vi "Init.vi"(8 "error in (no error)":errorcluster, 10 "Address":string, 11 "BPC30x in":refnum<class "BPC30x.lvclass">) -> (0 "error out":errorcluster, 3 "BPC30x out":refnum<class "BPC30x.lvclass">)   [LabVIEW 2023, in "BPC30x.lvlib" / "BPC30x.lvclass"]
uses:
  BPC30x.lvclass
  C:/Users/quantum/Documents/LVDAQ/UIs/TranslationStage_UI/Thorlabs.MotionControl.Controls.dll
  UIs/TranslationStage_UI/Thorlabs.MotionControl.Controls.dll
  typedefs/instrumentType.ctl
  typedefs/typedefs.lvlib
  <vilib>/ActorFramework/Actor/Actor.lvclass
  Interfaces/InitDeinitInterface/InitDeinitComm Messages/InitDone Msg/InitDone Msg.lvclass
  C:/Program Files/National Instruments/LabVIEW 2023/vi.lib/ActorFramework/Actor/Actor.lvclass
  C:/Users/quantum/Documents/LVDAQ/ConcreteClasses/ConcreteInstrumentClasses/BPC301/BPC30x/BPC30x.lvclass
  C:/Users/quantum/Documents/LVDAQ/Interfaces/InitDeinitInterface/InitDeinit/InitDeinit.lvclass
  C:/Users/quantum/Documents/LVDAQ/Interfaces/AbstractInstrumentClasses/TranslationStages_LV/TranslationStageInterface/TranslationStagesInterface.lvclass
  C:/Users/quantum/Documents/LVDAQ/UIs/TranslationStage_UI/Thorlabs.MotionControl.Benchtop.PiezoCLI.dll
  UIs/TranslationStage_UI/Thorlabs.MotionControl.Benchtop.PiezoCLI.dll
  <vilib>/ActorFramework/Message Enqueuer/Message Enqueuer.lvclass
panel:
  in  "BenchtopPiezoControl":refnum<k24>(container)
  out "BPC Enqueuer":refnum<class "Message Enqueuer.lvclass">
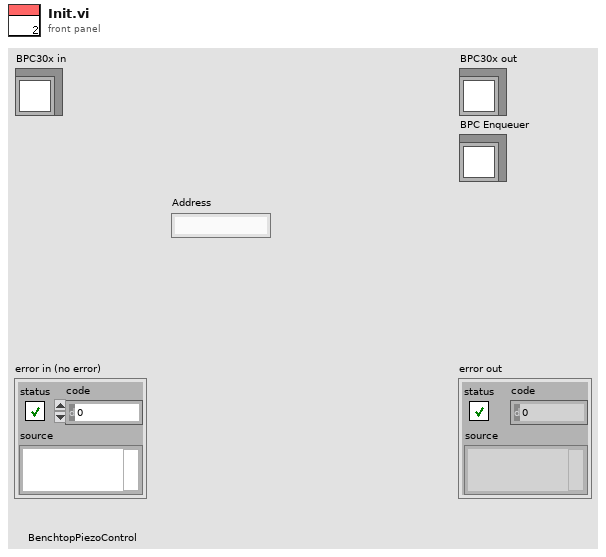
[diagram p1: front panel]
types:
  T1 = typedef "typedefs.lvlib/instrumentType.ctl" = enum16{"Spectrometer", "Camera", "Stepper", "Piezo"}
  T2 = cluster{"Output Voltage":dbl, "Channel Count":i32}
  T3 = cluster{"address type":enum16{"VISA", "Index"}, "Address":string, "instrument type":T1}
  T4 = cluster{"Instr Error":errorcluster, "Stepper Data":cluster{"Output Voltage":dbl, "Channel Count":i32}, "Address":cluster{"address type":enum16{"VISA", "Index"}, "Address":string, "instrument type":T1}}
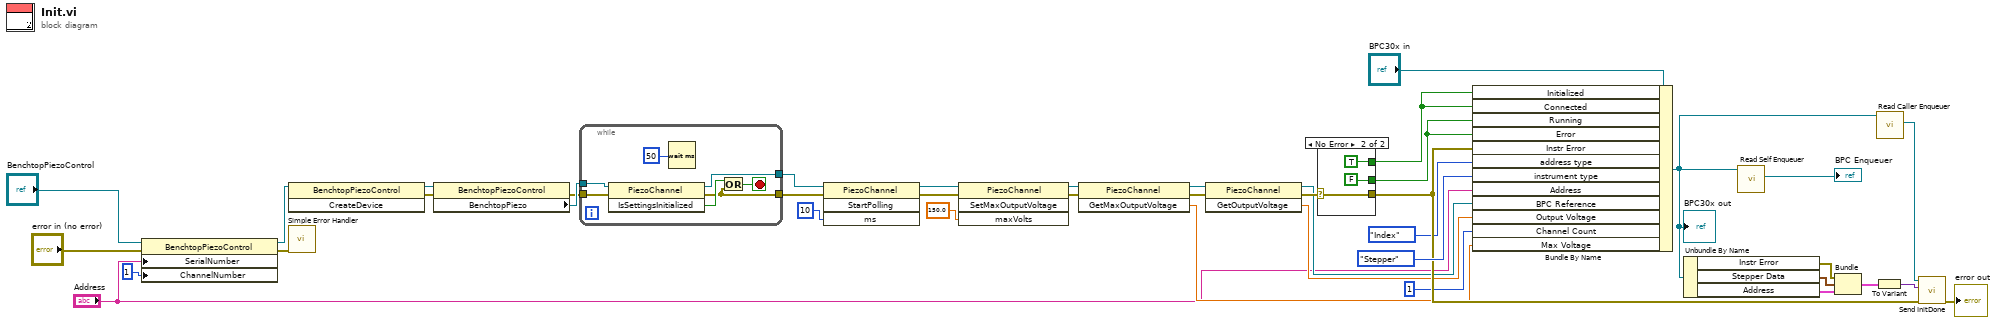
[diagram p0: block diagram]
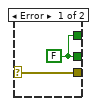
[diagram p2: hidden frame]
diagram:
  n1 = property class="BenchtopPiezoControl"(reference="BenchtopPiezoControl", error in="error in (no error)", "SerialNumber"="Address", "ChannelNumber"=1) -> (reference out=w31:refnum<k24>, error out=w28:errorcluster)
  n2 = invoke class="BenchtopPiezoControl" method="CreateDevice"(reference=w31) -> (reference out=w30:refnum<k24>, error out=w26:errorcluster)  [unwired: 2 in, 1 out]
  n3 = call <vilib>:"Simple Error Handler.vi"("error in (no error)"=w28) -> ()  [unwired: 4 in, 5 out]
  n4 = property class="BenchtopPiezoControl"(reference=w30, error in=w26) -> (error out=w25:errorcluster, "BenchtopPiezo"=w29:refnum<k24>)  [unwired: 1 out]
  n5 = while {
    tunnel: [w47] -> w17
    tunnel: [w44] -> w7
    tunnel: w29 -> [w41]
    tunnel: w25 -> [w42]
    stop <- w43 stop-if-true
    n6 = invoke class="PiezoChannel" method="IsSettingsInitialized"(reference=w41, error in=w42) -> (reference out=w47:refnum<k24>, error out=w44:errorcluster, "IsSettingsInitialized"=w45:bool)  [unwired: 1 in]
    n7 = Wait (ms)(milliseconds to wait=u32 50) -> ()  [unwired: 1 out]
    n8 = Or(x=w45, y=w44) -> (x .or. y?=w43:bool)
  }
  n9 = invoke class="PiezoChannel" method="StartPolling"(reference=w17, error in=w7, "ms"=10) -> (reference out=w12:refnum<k24>, error out=w8:errorcluster)  [unwired: 1 in, 2 out]
  n10 = invoke class="PiezoChannel" method="SetMaxOutputVoltage"(reference=w12, error in=w8, "maxVolts"=150.0) -> (reference out=w9:refnum<k24>, error out=w5:errorcluster)  [unwired: 1 in, 2 out]
  n11 = invoke class="PiezoChannel" method="GetMaxOutputVoltage"(reference=w9, error in=w5) -> (reference out=w11:refnum<k24>, error out=w6:errorcluster, "GetMaxOutputVoltage"=w10:dbl)  [unwired: 1 in]
  n12 = invoke class="PiezoChannel" method="GetOutputVoltage"(reference=w11, error in=w6) -> (reference out=w15:refnum<k24>, error out=w23:errorcluster, "GetOutputVoltage"=w19:dbl)  [unwired: 1 in]
  n13 = case shown="No Error" w23 {
    selector: w23 -> [w49 w52]
    tunnel: [w49 w52] -> w20
    tunnel: [w48 TRUE ("InstrumentData.CurrentState.Initialized")] -> w22
    tunnel: [w48 FALSE ("InstrumentData.CurrentState.Error")] -> w21
    frame Error {
      w48 = FALSE ("InstrumentData.CurrentState.Initialized")
    }
    frame No Error {
    }
  }
  n14 = Bundle By Name(cluster="BPC30x in", "Initialized"=w22, "Connected"=w22, "Running"=w21, "Error"=w21, "Instr Error"=w20, "address type"=enum16{"VISA", "Index"}."Index" ("InstrumentData.Address.address type"), "instrument type"=instrumentType."Stepper" ("InstrumentData.Address.instrument type"), "Address"="Address", "BPC Reference"=w15, "Output Voltage"=w19, "Channel Count"=1 ("Data.Channel Count"), "Max Voltage"=w10) -> (w14:refnum<class "BPC30x.lvclass">)
  "BPC30x out" <- w14
  n15 = Unbundle By Name(w14) -> ("Instr Error"=w35:errorcluster, "Stepper Data"=w36:T2, "Address"=w37:T3)
  n16 = call <vilib>:"Read Self Enqueuer.vi"("Actor"=w14) -> ("Self Enqueuer"=→"BPC Enqueuer":refnum<class "Message Enqueuer.lvclass">)  [unwired: 10 in]
  n17 = Bundle("Instr Error"=w35, "Stepper Data"=w36, "Address"=w37) -> (w38:T4)  [unwired: 1 in]
  n18 = call <vilib>:"Read Caller Enqueuer.vi"("Actor"=w14) -> ("Caller Enqueuer"=w34:refnum<class "Message Enqueuer.lvclass">)  [unwired: 10 in]
  n19 = To Variant(anything=w38) -> (Variant=w39:variant)
  n20 = call "Send InitDone.vi"("error in (no error)"=w20, "Variant"=w39, "Message Enqueuer"=w34) -> ("error out"=→"error out":errorcluster)  [unwired: 7 in, 1 out]
